vi "Test Merge.vi"() -> ()   [LabVIEW 2019, in "Instrument.Lockin.lvlib" / "Instrument.DAQ.lvclass"]
uses:
  Instrument.DAQ.lvclass
  <vilib>/LabVIEW Open Source Project/Data Manipulation/Variant/OpenVariant.lvlib
panel:
  out "element names":string[](array[string])
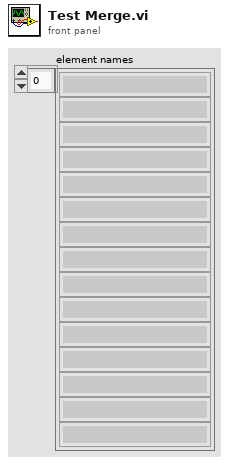
[diagram p1: front panel]
types:
  T1 = typedef "Instrument.Lockin.lvlib/Instrument.DAQ.lvclass/PublicEvents--Cluster.ctl" = cluster{"getAIChannels":refnum<user-event>, "getAOChannels":refnum<user-event>, "getREFChannels":refnum<user-event>, "getWaveforms":refnum<user-event>, "getResults":refnum<user-event>, "getSweepWaveforms":refnum<user-event>, "getCalibration":refnum<user-event>, "getDAQState":refnum<user-event>, "getDAQconfig":refnum<user-event>, "getInputGain":refnum<user-event>, "getOutputGain":refnum<user-event>, "getInputOffset":refnum<user-event>, "getSampling":refnum<user-event>, "getSweepChannels":refnum<user-event>, "getDeviceIDN":refnum<user-event>}
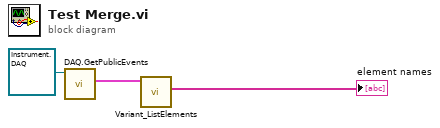
[diagram p0: block diagram]
diagram:
  n1 = call "DAQ.GetPublicEvents.vi"("Instrument.DAQ"=refnum<class "Instrument.DAQ.lvclass"> refnum) -> ("DAQ Public Events"=w2:T1)  [unwired: 8 in, 2 out]
  n2 = call <vilib>:"Variant_ListElements.vi"("Variant"=w2) -> ("element names"=→"element names":string[])  [unwired: 7 in, 3 out]
